vi "DPCal-Compute Max SPL.vi"(0 "Acoustic System":string, 1 "freqs":dbl[](array[numeric]), 2 "Attenuation (dB)":dbl[](array[numeric]), 5 "Probe mic gain (dB)":dbl, 7 "df (kHz)":dbl, 9 "Magnitude":dbl[](array[numeric]), 11 "error in (no error)":errorcluster) -> (4 "Max SPL1":dbl, 6 "Max SPL2":dbl, 15 "error out":errorcluster)   [LabVIEW 2020]
uses:
  cb8e5090-5c75-46f3-a9d5-d0e50d2f8b28.vi
  1fc9db3b-0123-488c-bb6f-0f171197ad53.vi
  fd590761-a5ef-4e95-bf37-9771a4973753.vi
  452da0ff-1ac1-4f8e-8ba4-370e78b8927d.vi
  epl-cal-vi-lib/Common VIs/Typedefs/CAL-Globals.vi
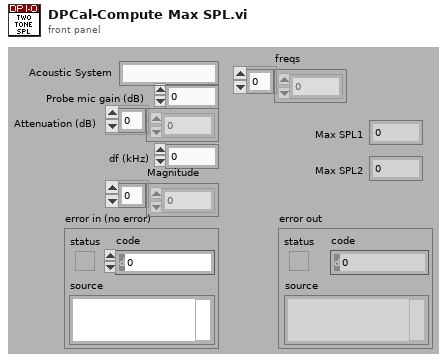
[diagram p1: front panel]
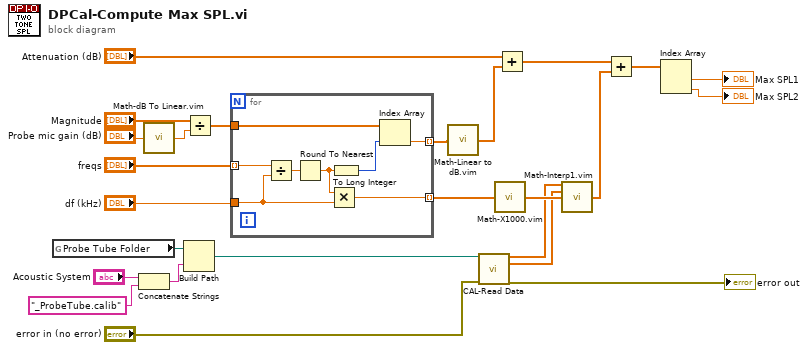
[diagram p0: block diagram]
diagram:
  n1 = global read "CAL-Globals.vi" "Probe Tube Folder"() -> (w9:path)
  n2 = Concatenate Strings("Acoustic System", "_ProbeTube.calib" ("string")) -> (w10:string)
  n3 = call "Math-dB To Linear.vim"("dB"="Probe mic gain (dB)") -> ("linear"=w21:dbl)
  n4 = Build Path(base path=w9, name or relative path=w10) -> (appended path=w7:path)
  n5 = Divide(x="Magnitude", y=w21) -> (x/y=w22:dbl[])
  n6 = for {
    tunnel: "df (kHz)" -> [w28]
    tunnel: "freqs" -> [w33] mode=indexing
    tunnel: w22 -> [w31]
    tunnel: [w26] -> w1 mode=indexing
    tunnel: [w27] -> w19 mode=indexing
    n7 = Divide(x=w33, y=w28) -> (x/y=w32:dbl)
    n8 = Round To Nearest(number=w32) -> (nearest integer value=w29:dbl)
    n9 = Multiply(x=w29, y=w28) -> (x*y=w27:dbl)
    n10 = To Long Integer(number=w29) -> (32bit integer=w30:i32)
    n11 = Index Array(array=w31, index=w30) -> (element=w26:dbl)
  }
  n12 = call "Math-Linear to dB.vim"("linear"=w1) -> ("dB"=w16:dbl[])
  n13 = call "CAL-Read Data.vi"("user path"=w7, "error in (no error)"="error in (no error)") -> ("Frequency (Hz)"=w6:dbl[], "Mag"=w5:dbl[], "error out"=→"error out":errorcluster)  [unwired: 9 in, 2 out]
  n14 = call "Math-X1000.vim"("X"=w19) -> ("1000X"=w12:dbl[])
  n15 = Add(x="Attenuation (dB)", y=w16) -> (x+y=w17:dbl[])
  n16 = call "Math-Interp1.vim"("X"=w6, "Y"=w5, "U"=w12) -> ("V"=w18:dbl[])  [unwired: 12 in]
  n17 = Add(x=w17, y=w18) -> (x+y=w13:dbl[])
  n18 = Index Array(array=w13) -> (element #1=→"Max SPL1":dbl, element #2=→"Max SPL2":dbl)  [unwired: 2 in]
